vi "视觉浏览器2.vi"() -> ()   [LabVIEW 2018]
uses:
  <vilib>/vision/NI_Vision_Development_Module.lvlib
panel:
  in  "布尔":bool
  out "error out":errorcluster
  out "Image":T1(plugin-control)
  in  "路径":path
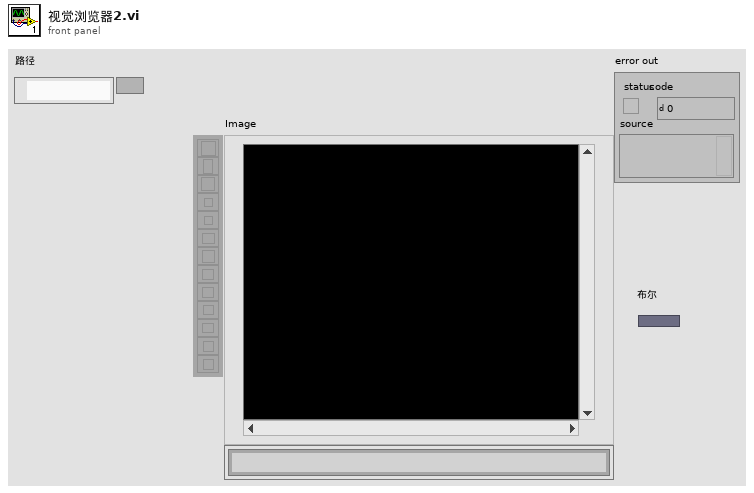
[diagram p1: front panel]
types:
  T1 = typedef "IMAQ Image.ctl" = refnum<image>
  T2 = typedef "Image Type" = u32
  T3 = cluster{"Browser Size":cluster{"X":i32, "Y":i32}, "Images per Line":i32, "Background Color":u32, "Frame Size":i32, "Frame Style":enum16{"Raised", "Bevelled", "Outline", "Hidden", "Step", "Raised Outline"}}
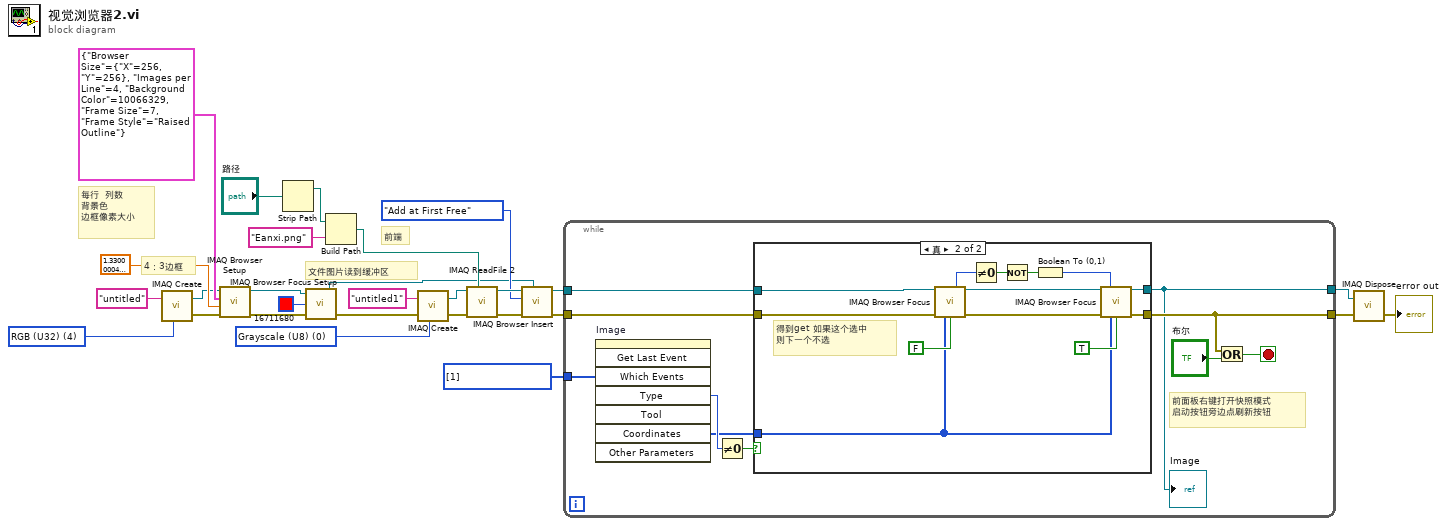
[diagram p0: block diagram]
diagram:
  w4 = i32[] [1] items=["No Event"=0, "Click Event"=1, "Draw Event"=2, "Size Event"=4, "Scroll Event"=5, "Double Click Event"=8] ("Which Events")
  w16 = T2 0 items=["Grayscale (U8)", "Grayscale (I16)", "Grayscale (SGL)", "Complex (CSG)", "RGB (U32)", "HSL (U32)", "RGB (U64)", "Grayscale (U16)"] ("Image Type")
  w26 = T2 4 items=["Grayscale (U8)", "Grayscale (I16)", "Grayscale (SGL)", "Complex (CSG)", "RGB (U32)", "HSL (U32)", "RGB (U64)", "Grayscale (U16)"] ("Image Type")
  # "每行  列数\n背景色\n边框像素大小"
  # "前端"
  # "文件图片读到缓冲区"
  # "4：3边框"
  n1 = call "IMAQ Create"("Image Name"="untitled", "Image Type"=w26) -> ("New Image"=w24:T1, "error out"=w23:errorcluster)  [unwired: 3 in]
  n2 = call "IMAQ Browser Setup"("error in (no error)"=w23, "Image Ratio"=sgl 1.33, "Browser Info"=T3 {"Browser Size"={"X"=256, "Y"=256}, "Images per Line"=4, "Background Color"=10066329, "Frame Size"=7, "Frame Style"=enum."Raised Outline"}, "Image In"=w24) -> ("error out"=w9:errorcluster, "Image Browser Out"=w10:T1)  [unwired: 2 out]
  n3 = Strip Path(path="路径") -> (stripped path=w21:path)  [unwired: 1 out]
  n4 = call "IMAQ Browser Focus Setup"("error in (no error)"=w9, "Focus Color"=u32 16711680, "Image Browser In"=w10) -> ("error out"=w6:errorcluster, "Image Browser Out"=w7:T1)  [unwired: 1 in]
  n5 = Build Path(base path=w21, name or relative path="Eanxi.png" ("名称或相对路径")) -> (appended path=w15:path)
  n6 = call "IMAQ Create"("Image Name"="untitled1", "Image Type"=w16, "error in (no error)"=w6) -> ("New Image"=w19:T1, "error out"=w17:errorcluster)  [unwired: 2 in]
  n7 = call "IMAQ ReadFile 2"("File Path"=w15, "error in (no error)"=w17, "Image"=w19) -> ("error out"=w13:errorcluster, "Image Out"=w14:T1)  [unwired: 4 in, 3 out]
  n8 = call "IMAQ Browser Insert"("Image Browser In"=w7, "error in (no error)"=w13, "Insertion Mode"=enum16{"Add at First Free", "Add at the End"}."Add at First Free", "Image to Add"=w14) -> ("error out"=w5:errorcluster, "Image Browser Out"=w3:T1)  [unwired: 3 in, 3 out]
  n9 = while {
    tunnel: w5 -> [w29]
    tunnel: w4 -> [w38]
    tunnel: w3 -> [w34]
    tunnel: [w30] -> w2
    tunnel: [w33] -> w1
    stop <- w31 stop-if-true
    # "前面板右键打开快照模式\n启动按钮旁边点刷新按钮"
    n10 = invoke on="Image" class="ImageControl" method="Get Last Event"("Which Events"=w38) -> ("Type"=w37:i32, "Coordinates"=w35:i32[])  [unwired: 7 in, 6 out]
    n11 = Not Equal To 0?(x=w37) -> (x != 0?=w36:bool)
    n12 = case shown="真" w36 {
      tunnel: w35 -> [_ w46]
      tunnel: w34 -> [w40 w52]
      tunnel: [w40 w43] -> w30
      tunnel: [w39 w42] -> w33
      tunnel: w29 -> [w39 w41]
      frame False {
      }
      frame True {
        # "得到get 如果这个选中\n则下一个不选"
        n13 = call "IMAQ Browser Focus"("Image Browser In"=w52, "error in (no error)"=w41, "Pixel Position"=w46, "Get/Set (Set)"=FALSE) -> ("State Out"=w51:enum16{"Not selected", "Selected"}, "Image Browser Out"=w44:T1, "error out"=w45:errorcluster)  [unwired: 6 in, 3 out]
        n14 = Not Equal To 0?(x=w51) -> (x != 0?=w50:bool)
        n15 = Not(x=w50) -> (.not. x?=w49:bool)
        n16 = Boolean To (0,1)(Boolean=w49) -> (0, 1=w48:i16)
        n17 = call "IMAQ Browser Focus"("Image Browser In"=w44, "State In"=w48, "error in (no error)"=w45, "Pixel Position"=w46, "Get/Set (Set)"=TRUE) -> ("Image Browser Out"=w43:T1, "error out"=w42:errorcluster)  [unwired: 5 in, 4 out]
      }
    }
    "Image" <- w30
    n18 = Or(x=w33, y="布尔") -> (x .or. y?=w31:bool)
  }
  n19 = call "IMAQ Dispose"("Image"=w2, "error in (no error)"=w1) -> ("error out"=→"error out":errorcluster)  [unwired: 4 in]
